vi "Register-user-events.vi"(8 "error in (no error)":errorcluster, 11 "Object ref in":T1) -> (0 "error out":errorcluster, 2 "Event registration":refnum<event-registration>, 3 "Object ref out":T1)   [LabVIEW 2013, in "SLMControl.lvlib" / "SC-Main.lvclass"]
uses:
  SC-Main.lvclass
  Object-reference.ctl
  SC-Main.lvclass/SC-Main.ctl
  Read Activity log.vi
  Read Error log.vi
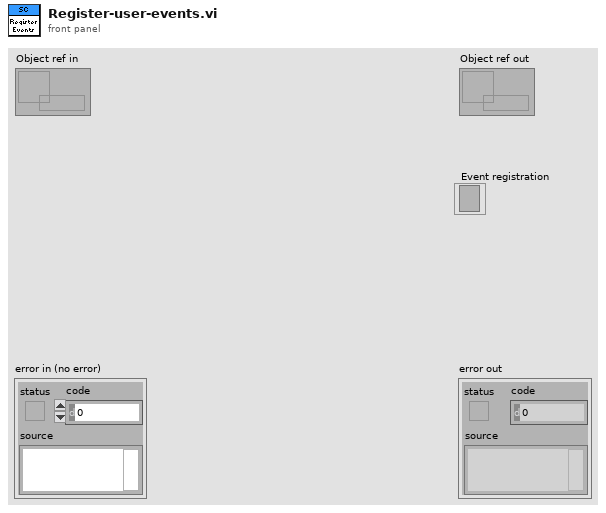
[diagram p1: front panel]
types:
  T1 = typedef "SLMControl.lvlib/SC-Main.lvclass/Object-reference.ctl" = refnum<data-value>
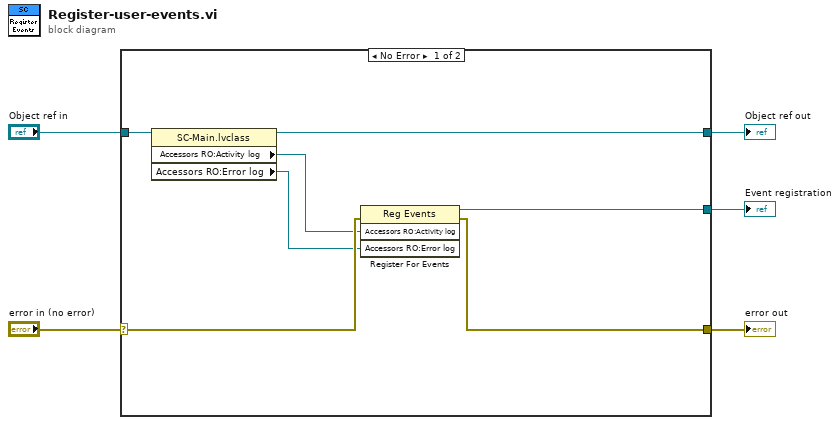
[diagram p0: block diagram]
diagram:
  n1 = case shown="No Error" "error in (no error)" {
    selector: "error in (no error)" -> [w10 w14]
    tunnel: [w9 w14] -> w4
    tunnel: [w11 w13] -> w2
    tunnel: "Object ref in" -> [w12 w13]
    tunnel: [w6 _] -> w1
    frame No Error {
      n2 = property class="SC-Main.lvclass"(reference=w12) -> (reference out=w11:T1, "Accessors RO:Activity log"=w8:refnum<user-event>, "Accessors RO:Error log"=w7:refnum<user-event>)  [unwired: 1 in, 1 out]
      n3 = register-events(error in=w10, w8, w7) -> (reference out=w6:refnum<event-registration>, error out=w9:errorcluster)  [unwired: 1 in]
    }
    frame Error {
    }
  }
  "error out" <- w4
  "Object ref out" <- w2
  "Event registration" <- w1
